vi "Set wavegen DC signal parameters.vi"(7 "Load Impedance":T2, 8 "error in (no error)":errorcluster {"code" format="%.0x"}, 9 "DC Voltage level":dbl, 11 "instrument handle in":refnum<k15>) -> (0 "error out":errorcluster, 2 "log string out":string, 3 "instrument handle out":refnum<k15>)   [LabVIEW 2017]
uses:
  Load Impedance.ctl
  Waveform type.ctl
  <instrlib>/Keysight InfiniiVision/Keysight InfiniiVision.lvlib
panel:
  out "*(type *) &x":T1
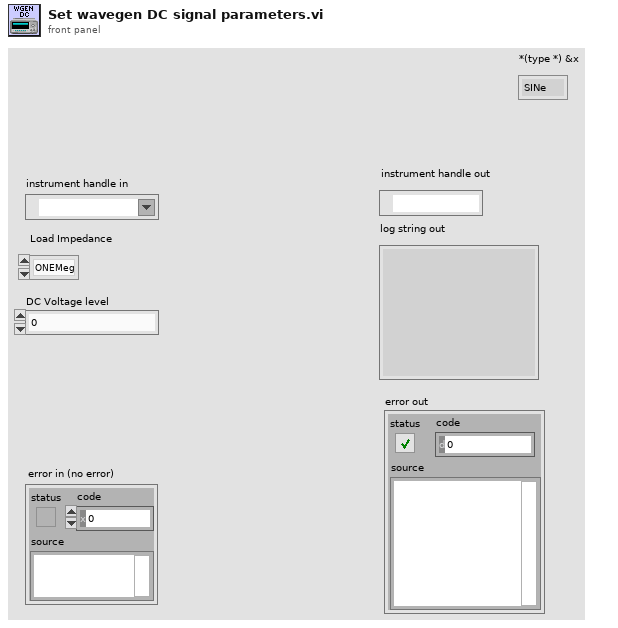
[diagram p1: front panel]
types:
  T1 = typedef "Waveform type.ctl" = enum16{"SINe", "SQUare", "RAMP", "PULSe", "DC", "NOISe"}
  T2 = typedef "Load Impedance.ctl" = enum16{"ONEMeg", "FIFTy"}
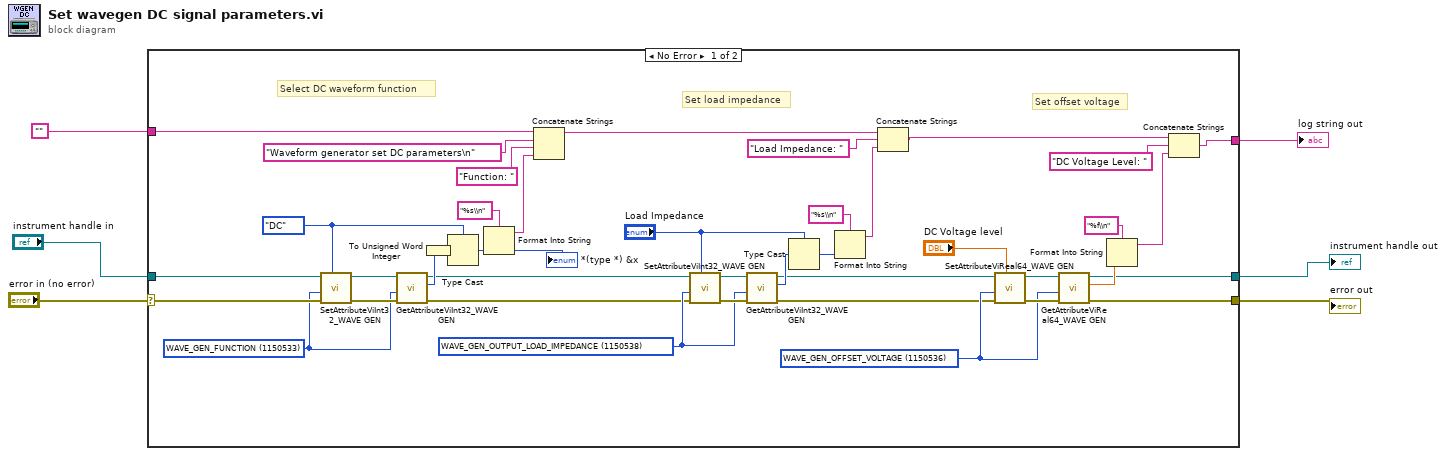
[diagram p0: block diagram]
diagram:
  n1 = case shown="No Error" "error in (no error)" {
    selector: "error in (no error)" -> [w45 w47]
    tunnel: "instrument handle in" -> [w46 w48]
    tunnel: [w29 w48] -> w2
    tunnel: [w28 w47] -> w1
    tunnel: [w27 w49] -> w3
    tunnel: "" ("log string in") -> [w25 w49]
    frame No Error {
      w21 = u32 1150538 items=["ARBITRARY_BYTE_ORDER"=1150415, "MODULATION_FUNCTION"=1150552, "MODULATION_TYPE"=1150555, "TRACKING_PHASE"=1150659, "WAVE_GEN_ADDITIONAL_NOISE"=1150529, "WAVE_GEN_ARBITRARY_BYTE_ORDER"=1150544, "WAVE_GEN_FUNCTION"=1150533, "WAVE_GEN_OUTPUT_LOAD_IMPEDANCE"=1150538, "WAVE_GEN_OUTPUT_MODE"=1150658] ("AttributeID")
      w24 = u32 1150536 items=["FM_DEVIATION"=1150548, "FM_FREQUENCY"=1150549, "FSK_FREQUENCY"=1150550, "FSK_MODULATION_RATE"=1150551, "MODULATION_RAMP_SYMMETRY"=1150553, "WAVE_GEN_AM_DEPTH"=1150546, "WAVE_GEN_AM_FREQUENCY"=1150547, "WAVE_GEN_AMPLITUDE"=1150530, "WAVE_GEN_DUTY_CYCLE"=1150531, "WAVE_GEN_FREQUENCY"=1150532, "WAVE_GEN_HIGH_VOLTAGE"=1150534, "WAVE_GEN_LOW_VOLTAGE"=1150535, "WAVE_GEN_OFFSET_VOLTAGE"=1150536, "WAVE_GEN_PERIOD"=1150539, "WAVE_GEN_PULSE_WIDTH"=1150540, "WAVE_GEN_RAMP_SYMMETRY"=1150541] ("AttributeID")
      w40 = Waveform_type."DC"
      w42 = u32 1150533 items=["ARBITRARY_BYTE_ORDER"=1150415, "MODULATION_FUNCTION"=1150552, "MODULATION_TYPE"=1150555, "TRACKING_PHASE"=1150659, "WAVE_GEN_ADDITIONAL_NOISE"=1150529, "WAVE_GEN_ARBITRARY_BYTE_ORDER"=1150544, "WAVE_GEN_FUNCTION"=1150533, "WAVE_GEN_OUTPUT_LOAD_IMPEDANCE"=1150538, "WAVE_GEN_OUTPUT_MODE"=1150658] ("AttributeID")
      # "Set load impedance"
      # "Set offset voltage"
      # "Select DC waveform function"
      n2 = call <instrlib>:"SetAttributeViInt32_WAVE GEN.vi"("AttributeValue"=w40, "error in (no error)"=w45, "AttributeID"=w42, "instrument handle"=w46) -> ("error out"=w43:errorcluster, "instrument handle out"=w44:refnum<k15>)  [unwired: 6 in]
      n3 = call <instrlib>:"GetAttributeViInt32_WAVE GEN.vi"("error in (no error)"=w43, "AttributeID"=w42, "instrument handle"=w44) -> ("error out"=w15:errorcluster, "AttributeValue"=w41:i32, "instrument handle out"=w16:refnum<k15>)  [unwired: 6 in]
      n4 = To Unsigned Word Integer(number=w41) -> (unsigned 16bit integer=w7:u16)
      n5 = Type Cast(type=w40, x=w7) -> (*(type *) &x=w39:T1)
      "*(type *) &x" <- w39
      n6 = Format Into String(format string="%s\\n", w39) -> (resulting string=w38:string)  [unwired: 2 in, 1 out]
      n7 = Concatenate Strings(w25, "Waveform generator set DC parameters\n" ("string"), "Function: " ("string"), w38) -> (w12:string)
      n8 = call <instrlib>:"SetAttributeViInt32_WAVE GEN.vi"("AttributeValue"="Load Impedance", "error in (no error)"=w15, "AttributeID"=w21, "instrument handle"=w16) -> ("error out"=w23:errorcluster, "instrument handle out"=w22:refnum<k15>)  [unwired: 6 in]
      n9 = call <instrlib>:"GetAttributeViInt32_WAVE GEN.vi"("error in (no error)"=w23, "AttributeID"=w21, "instrument handle"=w22) -> ("error out"=w9:errorcluster, "AttributeValue"=w19:i32, "instrument handle out"=w10:refnum<k15>)  [unwired: 6 in]
      n10 = Type Cast(type="Load Impedance", x=w19) -> (*(type *) &x=w14:T2)
      n11 = Format Into String(format string="%s\\n", w14) -> (resulting string=w17:string)  [unwired: 2 in, 1 out]
      n12 = Concatenate Strings(w12, "Load Impedance: " ("string"), w17) -> (w11:string)
      n13 = call <instrlib>:"SetAttributeViReal64_WAVE GEN.vi"("AttributeValue"="DC Voltage level", "error in (no error)"=w9, "AttributeID"=w24, "instrument handle"=w10) -> ("error out"=w34:errorcluster, "instrument handle out"=w35:refnum<k15>)  [unwired: 6 in]
      n14 = call <instrlib>:"GetAttributeViReal64_WAVE GEN.vi"("error in (no error)"=w34, "AttributeID"=w24, "instrument handle"=w35) -> ("error out"=w28:errorcluster, "AttributeValue"=w30:dbl, "instrument handle out"=w29:refnum<k15>)  [unwired: 6 in]
      n15 = Format Into String(format string="%f\\n", w30) -> (resulting string=w31:string)  [unwired: 2 in, 1 out]
      n16 = Concatenate Strings(w11, "DC Voltage Level: " ("string"), w31) -> (w27:string)
    }
    frame Error {
    }
  }
  "log string out" <- w3
  "instrument handle out" <- w2
  "error out" <- w1
